vi "String - Find IP MAC and Model Number from ProtoBuf String.vi"(8 "error in":errorcluster, 11 "Decoded ProtoBuf Mesage In":string="msg_time_stamp: 1881779473\r\npwr_status: 4\r\nbatt_status: 100\r\nanalog_in_port_num: 16\r\nanalog_in_port_num_priv: 8\r\nanalog_in_port_av_range: 5\r\nanalog_in_res: 4096\r\nanalog_in_res_priv: 4096\r\ndigital_port_num: 16\r\nip_addr: \"\\300\\250\\001\\001\"\r\nnet_mask: \"\\377\\377\\377\\000\"\r\ngateway: \"\\300\\250\\001\\001\"\r\nprimary_dns: \"\\300\\250\\001\\001\"\r\nsecondary_dns: \"\\300\\250\\001\\001\"\r\nmac_addr: \"\\370\\360\\005\\244\\247\\301\"\r\nhost_name: \"NYQUIST\"\r\ndevice_port: 9760\r\ndevice_pn: \"Nq1\"\r\ndevice_hw_rev: \"2.0.0\"\r\ndevice_fw_rev: \"1.0.3\"\r\ndevice_sn: 9090668548463847645\r\n") -> (0 "error out":errorcluster, 1 "Model Number":string, 2 "MAC Address String":string, 3 "IP Address":string)   [LabVIEW 2020]
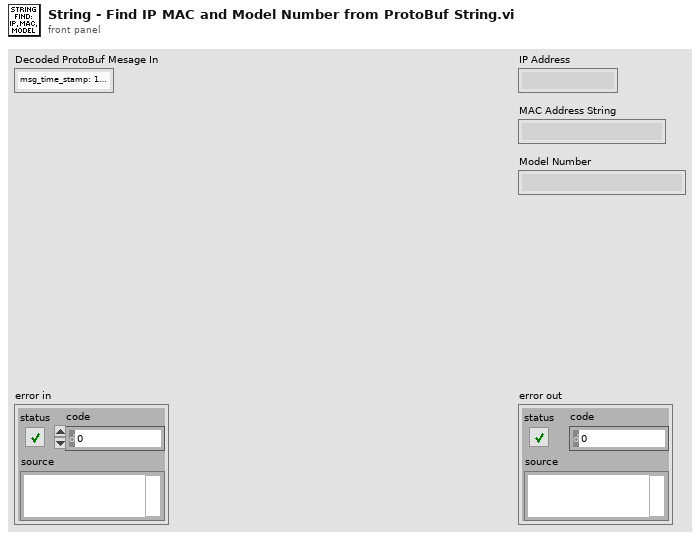
[diagram p1: front panel]
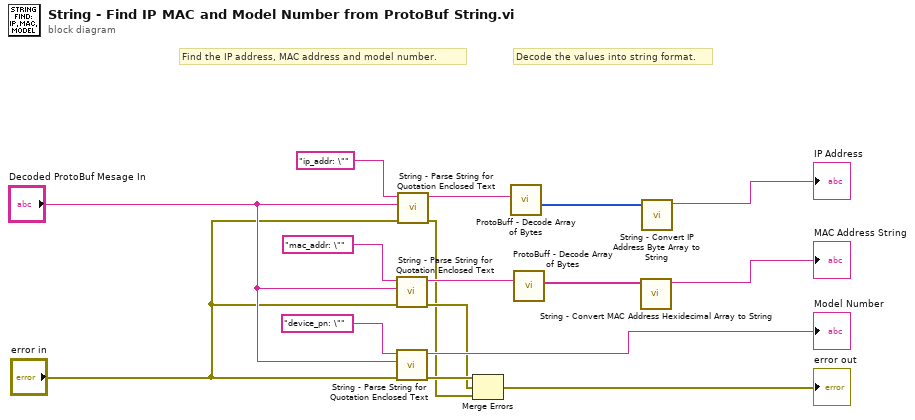
[diagram p0: block diagram]
diagram:
  # "Decode the values into string format."
  # "Find the IP address, MAC address and model number."
  n1 = call "String - Parse String for Quotation Enclosed Text.vi"("error in"="error in", "Input String"="Decoded ProtoBuf Mesage In", "Search String"="mac_addr: \"" ("search string")) -> ("error out"=w3:errorcluster, "result string"=w13:string)  [unwired: 7 in]
  n2 = call "String - Parse String for Quotation Enclosed Text.vi"("error in"="error in", "Input String"="Decoded ProtoBuf Mesage In", "Search String"="device_pn: \"" ("search string")) -> ("error out"=w4:errorcluster, "result string"=→"Model Number":string)  [unwired: 7 in]
  n3 = call "String - Parse String for Quotation Enclosed Text.vi"("error in"="error in", "Input String"="Decoded ProtoBuf Mesage In", "Search String"="ip_addr: \"" ("search string")) -> ("error out"=w2:errorcluster, "result string"=w15:string)  [unwired: 7 in]
  n4 = Merge Errors(w4, w3, w2) -> (→"error out":errorcluster)
  n5 = call "ProtoBuff - Decode Array of Bytes.vi"("Encoded String"=w15) -> ("Array of Bytes"=w10:u8[])  [unwired: 9 in, 1 out]
  n6 = call "ProtoBuff - Decode Array of Bytes.vi"("Encoded String"=w13) -> ("Hexidecimal Strings"=w8:string[])  [unwired: 9 in, 1 out]
  n7 = call "String - Convert MAC Address Hexidecimal Array to String.vi"("Hexidecimal Strings"=w8) -> ("MAC Address String"=→"MAC Address String":string)  [unwired: 10 in]
  n8 = call "String - Convert IP Address Byte Array to String.vi"("Array of Bytes"=w10) -> ("IP Address String"=→"IP Address":string)  [unwired: 10 in]
